vi "Get Logging Event.vi"(8 "error in":errorcluster, 11 "UserEventHandler in":refnum<class "UserEventHandler.lvclass">) -> (0 "error out":errorcluster, 2 "Logging Event":refnum<user-event>, 3 "UserEventHandler out":refnum<class "UserEventHandler.lvclass">)   [LabVIEW 2020, in "hse-logger.lvlib" / "UserEventHandler.lvclass"]
doc: "Returns the ``Logging Event`` from the object. This ``Logging Event`` can be registered in any Event Structure.\n\n____\nHAMPEL SOFTWARE ENGINEERING v2.0.6 (2021-04-15 11:38)"
uses:
  UserEventHandler.lvclass
  LogRecord/LogRecord.lvclass
  UserEventHandler.lvclass/UserEventHandler.ctl
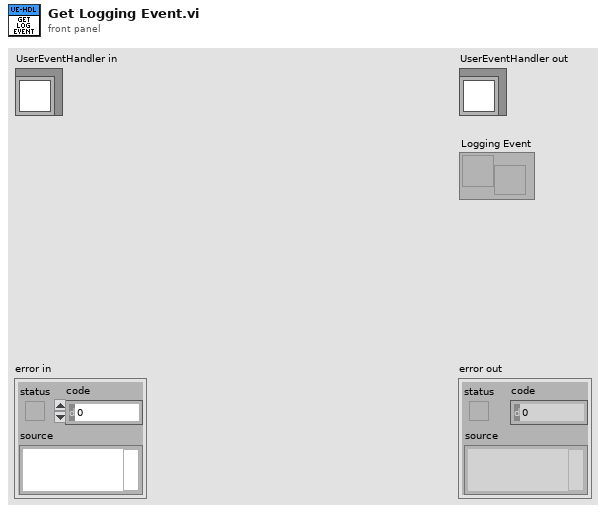
[diagram p1: front panel]
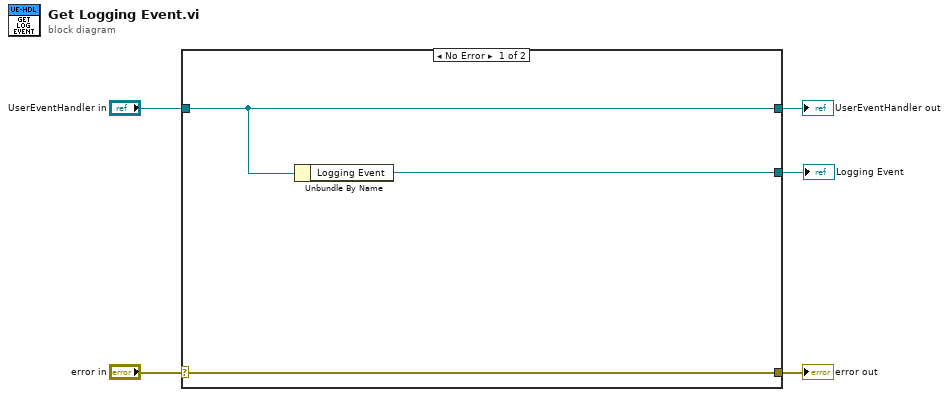
[diagram p0: block diagram]
diagram:
  n1 = case shown="No Error" "error in" {
    selector: "error in" -> [w8 w10]
    tunnel: [w8 w10] -> w4
    tunnel: [w7 w9] -> w2
    tunnel: "UserEventHandler in" -> [w7 w9]
    tunnel: [w6 _] -> w1
    frame No Error {
      n2 = Unbundle By Name(w7) -> ("Logging Event"=w6:refnum<user-event>)
    }
    frame Error {
    }
  }
  "error out" <- w4
  "UserEventHandler out" <- w2
  "Logging Event" <- w1
